vi "Command_TurretControl.vi"(0 "Shooter_Table":dbl[][](array[numeric])=[[55.0, 3350.0, 60.5], [81.0, 3500.0, 54.5], [110.0, 3800.0, 50.5], [143.0, 4100.0, 48.5], [179.0, 4700.0, 47.5], [220.0, 4800.0, 47.5], [250.0, 5800.0, 47.5], [280.0, 5800.0, 45.0]], 3 "Parameters":dbl[](array[numeric]), 6 "Startup":bool) -> (16 "Completed":bool, 17 "Reinit":bool, 20 "Turret_Control_State":T3=enum."No-Op", 21 "Turret_Goal_Angle":dbl, 22 "Camera_Goal_X (deg)":dbl, 23 "Flywheel_Control_State":T2=enum."Speed_Control", 24 "Passive Flywheel Velocity (RPM)":dbl=4000.0, 26 "Cowl_Control_State":T1=enum."No-Op", 27 "Target Cowl Angle (deg)":dbl=52.0)   [LabVIEW 2020]
uses:
  Subsystems/Turret/Turret_States.ctl
  Subsystems/Flywheel/Flywheel_States.ctl
  Subsystems/Cowl/Cowl_States.ctl
  Auto Utilities/Command_Execution_State.ctl
  Globals/Sensor_Values.vi
  Systems/Shooter/Determiner/Shooter_Globals.vi
  Globals/Turret_Globals.vi
panel:
  in  "Shooter_Table 2":dbl[][](array[numeric])=[[55.0, 3350.0, 60.5], [81.0, 3500.0, 54.5], [110.0, 3800.0, 50.5], [143.0, 4100.0, 48.5], [179.0, 4700.0, 47.5], [220.0, 4800.0, 47.5], [250.0, 5800.0, 47.5], [280.0, 5800.0, 45.0]]
  out "angle_to_target":dbl
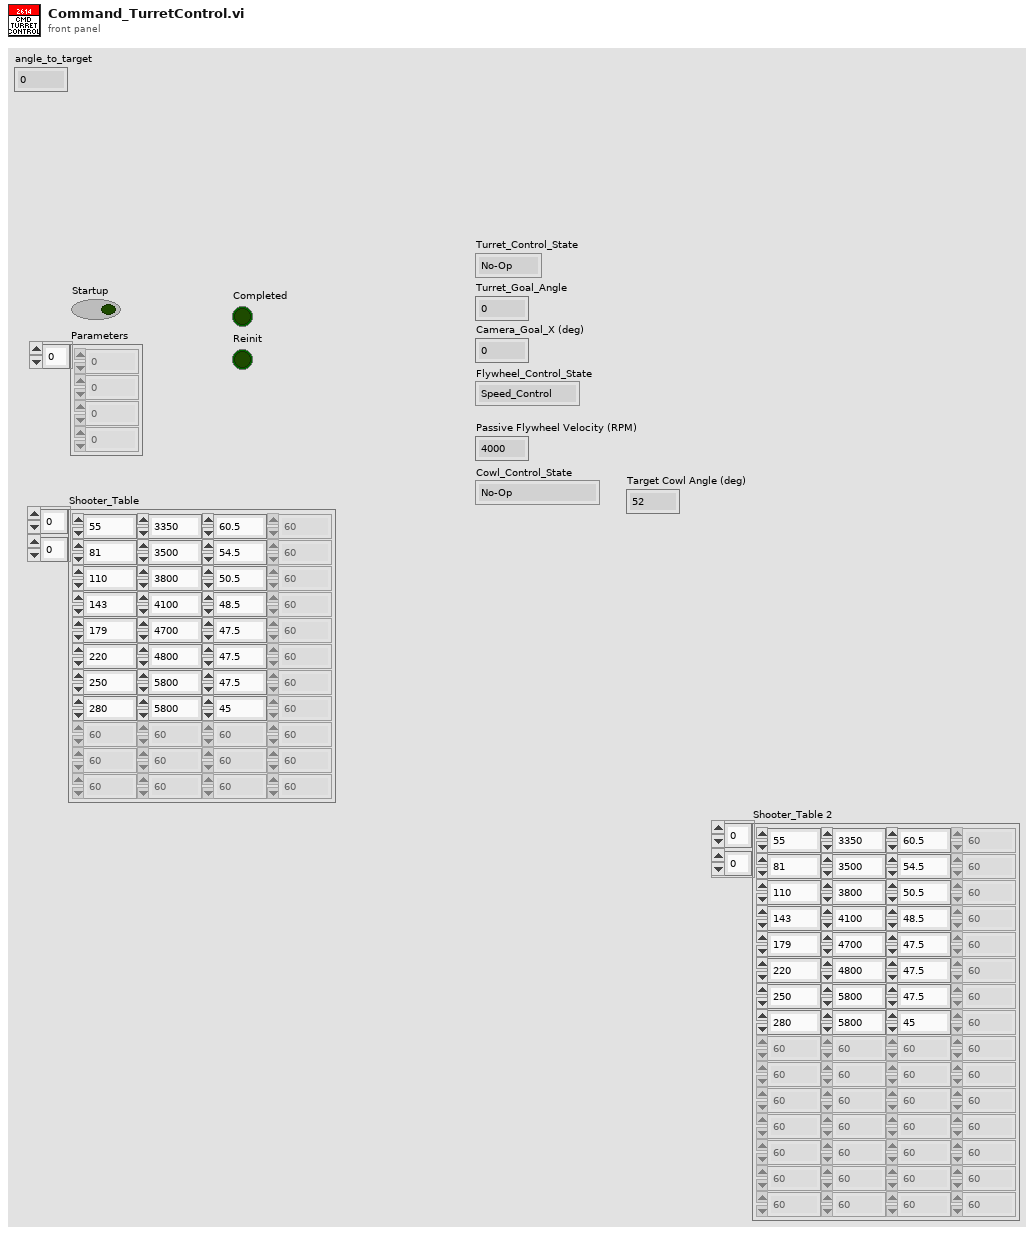
[diagram p1: front panel]
types:
  T1 = typedef "Cowl_States.ctl" = enum16{"Manual_%VBus", "GoToAngle", "No-Op", "GoToZero"}
  T2 = typedef "Flywheel_States.ctl" = enum16{"No-Op", "Percent_Voltage", "Speed_Control", "Speed_Control_Manual", "Command_SpinUp", "Command_SpinUpAuto"}
  T3 = typedef "Turret_States.ctl" = enum16{"Manual_Percent_Voltage", "Target_With_Limelight", "Command_TurnToPosition", "Command_Auto_Target", "GoToZero", "No-Op", "Test_Position_Control", "Position_Control"}
  T4 = typedef "Command_Execution_State.ctl" = enum16{"Initialize", "Execute", "Finish"}
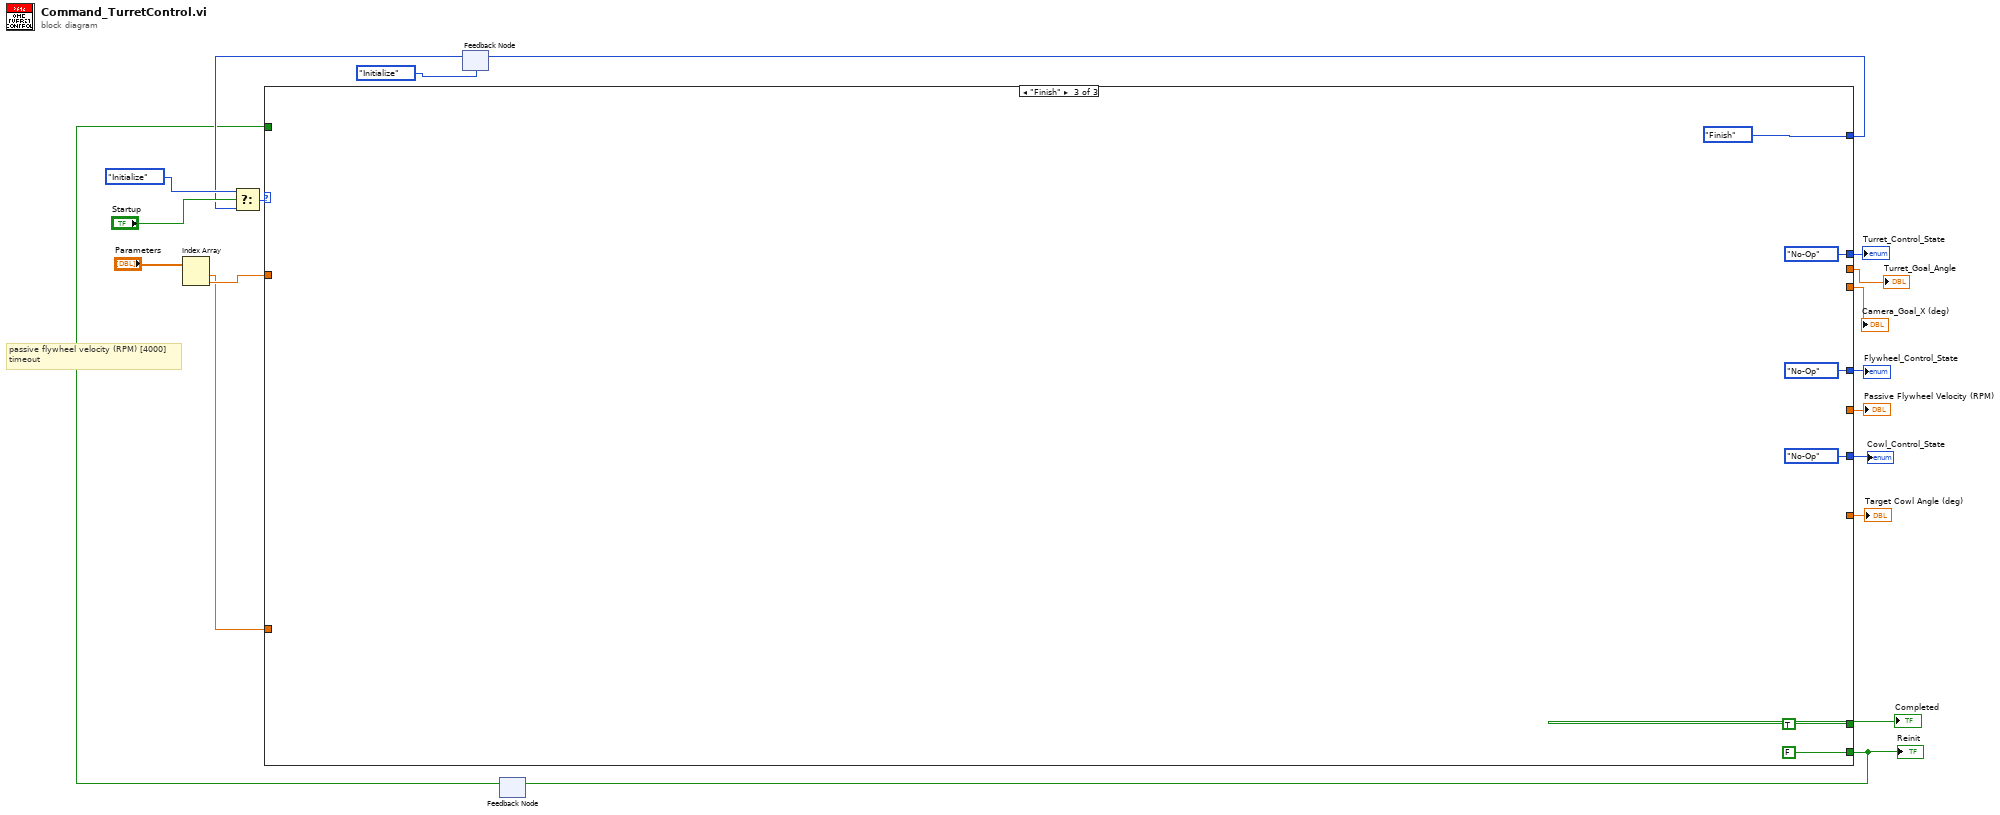
[diagram p0: block diagram]
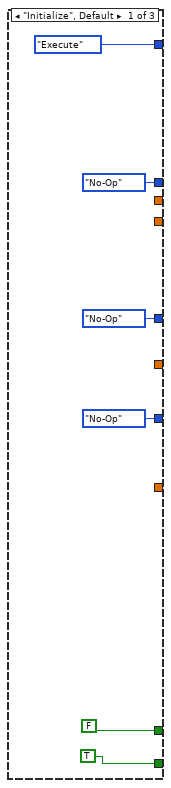
[diagram p2: hidden frame]
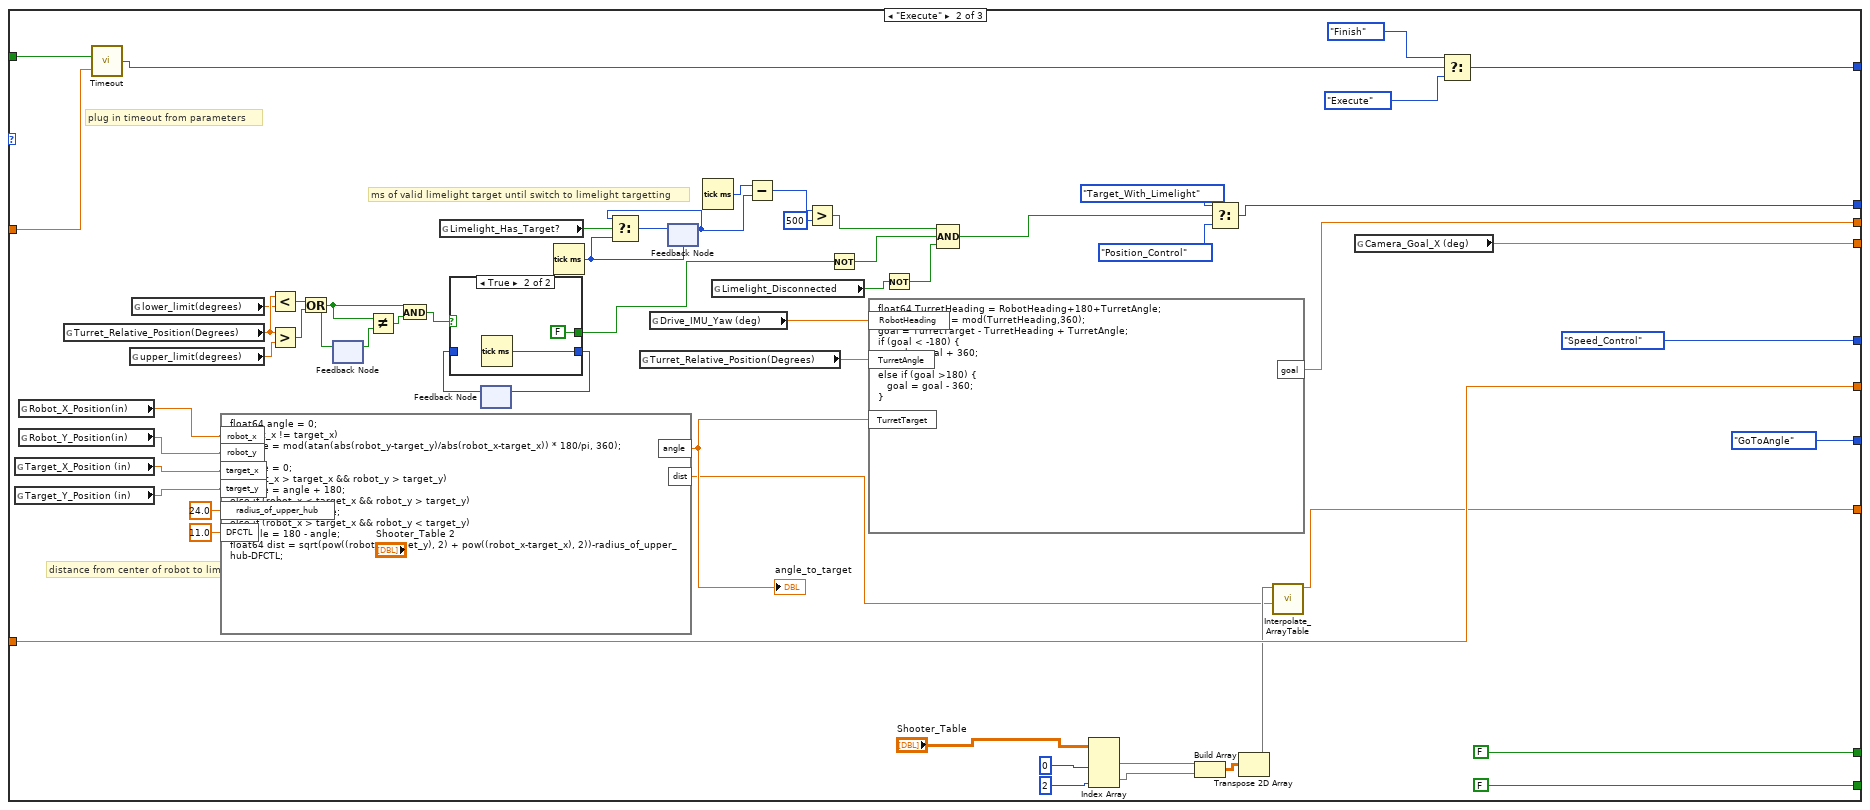
[diagram p3: hidden frame]
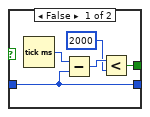
[diagram p4: hidden frame]
diagram:
  # "passive flywheel velocity (RPM) [4000]\ntimeout"
  n1 = Index Array(array="Parameters") -> (element #1=w3:dbl, element #2=w4:dbl)  [unwired: 2 in]
  n2 = feedback #1(Command_Execution_State."Initialize") -> (w15:T4)
  n3 = Select(t=Command_Execution_State."Initialize", s="Startup", f=w15) -> (s? t:f=w17:T4)
  n4 = feedback #2() -> (w11:bool)  [unwired: 1 in]
  n5 = case shown="\"Finish\"" w17 {
    tunnel: [Command_Execution_State."Execute" w81 Command_Execution_State."Finish"] -> w16
    tunnel: [FALSE ("Reinit") FALSE ("Reinit") TRUE ("Reinit")] -> w13
    tunnel: [TRUE ("Reinit") FALSE ("Reinit") FALSE ("Reinit")] -> w12
    tunnel: w11 -> [_ w78 _]
    tunnel: [Turret_States."No-Op" ("Control_State") w48 Turret_States."No-Op" ("Control_State")] -> w9
    tunnel: [_ w47 _] -> w7
    tunnel: [_ w46 _] -> w8
    tunnel: [_ w43 _] -> w6
    tunnel: [Flywheel_States."No-Op" ("Flywheel_Control_State") Flywheel_States."Speed_Control" ("Flywheel_Control_State") Flywheel_States."No-Op" ("Flywheel_Control_State")] -> w5
    tunnel: w4 -> [_ w44 _]
    tunnel: w3 -> [_ w43 _]
    tunnel: [Cowl_States."No-Op" ("Cowl_Control_State") Cowl_States."GoToAngle" ("Cowl_Control_State") Cowl_States."No-Op" ("Cowl_Control_State")] -> w2
    tunnel: [_ w26 _] -> w1
    frame "Initialize", Default {
    }
    frame "Execute" {
      # "distance from center of robot to limelight"
      # "ms of valid limelight target until switch to limelight targetting"
      # "plug in timeout from parameters"
      n6 = global read "Shooter_Globals.vi" "Target_X_Position (in)"() -> (w40:dbl)
      n7 = global read "Shooter_Globals.vi" "Target_Y_Position (in)"() -> (w39:dbl)
      n8 = global read "Sensor_Values.vi" "Robot_X_Position(in)"() -> (w42:dbl)
      n9 = global read "Sensor_Values.vi" "Robot_Y_Position(in)"() -> (w41:dbl)
      n10 = global read "Sensor_Values.vi" "Turret_Relative_Position(Degrees)"() -> (w54:dbl)
      n11 = call "Timeout.vi"("Timeout"=w44, "Initialize"=w78) -> ("Timed Out?"=w77:bool)
      n12 = global read "Turret_Globals.vi" "upper_limit(degrees)"() -> (w52:dbl)
      n13 = global read "Turret_Globals.vi" "lower_limit(degrees)"() -> (w51:dbl)
      n14 = formula code="float64 angle = 0;\nif(robot_x != target_x)\n    angle = mod(atan(abs(robot_y-target_y)/abs(robot_x-target_x)) * 180/pi, 360);\nelse\n    angle = 0;\nif (robot_x > target_x && robot_y > target_y)\n    angle = angle + 180;\nelse if (robot_x < target_x && robot_y > target_y)\n    angle = 360 - angle;\nelse if (robot_x > target_x && robot_y < target_y)\n    angle = 180 - angle;\nfloat64 dist = sqrt(pow((robot_y-target_y), 2) + pow((robot_x-target_x), 2))-radius_of_upper_hub-DFCTL;"("robot_x"=w42, "robot_y"=w41, "target_x"=w40, "target_y"=w39, "radius_of_upper_hub"=24.0 ("input variable"), "DFCTL"=11.0 ("input variable")) -> ("angle"=w36:dbl, "dist"=w28:dbl)
      "angle_to_target" <- w36
      n15 = Less?(x=w54, y=w51) -> (x < y?=w55:bool)
      n16 = Greater?(x=w54, y=w52) -> (0:w53:bool)
      n17 = Or(x=w55, y=w53) -> (x .or. y?=w56:bool)
      n18 = feedback #3() -> (w57:bool)  [unwired: 1 in]
      n19 = feedback-in #3(w56) -> ()
      n20 = Not Equal?(x=w56, y=w57) -> (x != y?=w58:bool)
      n21 = And(x=w56, y=w58) -> (x .and. y?=w59:bool)
      n22 = global read "Sensor_Values.vi" "Limelight_Has_Target?"() -> (w73:bool)
      n23 = feedback #4() -> (w65:u32)  [unwired: 1 in]
      n24 = case shown="True" w59 {
        tunnel: w65 -> [w88 _]
        tunnel: [w88 w90] -> w64
        tunnel: [w87 FALSE] -> w63
        frame False {
          n25 = Tick Count (ms)() -> (millisecond timer value=w85:u32)
          n26 = Subtract(x=w85, y=w88) -> (x-y=w86:u32)
          n27 = Less?(x=w86, y=u32 2000) -> (x < y?=w87:bool)
        }
        frame True {
          n28 = Tick Count (ms)() -> (millisecond timer value=w90:u32)
        }
      }
      n29 = feedback-in #4(w64) -> ()
      n30 = Tick Count (ms)() -> (millisecond timer value=w72:u32)
      n31 = global read "Sensor_Values.vi" "Turret_Relative_Position(Degrees)"() -> (w66:dbl)
      n32 = global read "Sensor_Values.vi" "Drive_IMU_Yaw (deg)"() -> (w67:dbl)
      n33 = feedback #5(w72) -> (w75:u32)
      n34 = Select(t=w75, s=w73, f=w72) -> (s? t:f=w74:u32)
      n35 = feedback-in #5(w74) -> ()
      n36 = Tick Count (ms)() -> (millisecond timer value=w71:u32)
      n37 = global read "Sensor_Values.vi" "Limelight_Disconnected"() -> (w50:bool)
      n38 = Subtract(x=w71, y=w75) -> (x-y=w76:u32)
      n39 = Greater?(x=w76, y=u32 500) -> (0:w60:bool)
      n40 = Not(x=w63) -> (.not. x?=w62:bool)
      n41 = formula code="float64 TurretHeading = RobotHeading+180+TurretAngle;\nTurretHeading = mod(TurretHeading,360);\ngoal = TurretTarget - TurretHeading + TurretAngle;\nif (goal < -180) {\n   goal = goal + 360;\n} \nelse if (goal >180) {\n   goal = goal - 360;\n}"("TurretAngle"=w66, "RobotHeading"=w67, "TurretTarget"=w36) -> ("goal"=w46:dbl)
      n42 = Not(x=w50) -> (.not. x?=w49:bool)
      n43 = Compound Arithmetic op=AND(w60, w62, w49) -> (w61:bool)
      n44 = Index Array(array="Shooter_Table", index (col) #1=0 ("index (row)"), index (col) #2=2 ("index (row)")) -> (element #1=w35:dbl[], element #2=w34:dbl[])  [unwired: 2 in]
      n45 = Build Array(w35, w34) -> (w31:dbl[][])
      n46 = Select(t=Turret_States."Target_With_Limelight" ("Control_State"), s=w61, f=Turret_States."Position_Control" ("Control_State")) -> (s? t:f=w48:T3)
      n47 = Transpose 2D Array(2D array=w31) -> (transposed array=w30:dbl[][])
      n48 = call "Interpolate_ArrayTable.vi"("Desired_Distance"=w28, "array"=w30) -> ("RPM"=w26:dbl)  [unwired: 9 in]
      n49 = global read "Sensor_Values.vi" "Camera_Goal_X (deg)"() -> (w47:dbl)
      n50 = Select(t=Command_Execution_State."Finish", s=w77, f=Command_Execution_State."Execute") -> (s? t:f=w81:T4)
    }
    frame "Finish" {
    }
  }
  "Reinit" <- w12
  "Completed" <- w13
  "Turret_Control_State" <- w9
  "Turret_Goal_Angle" <- w8
  "Camera_Goal_X (deg)" <- w7
  "Passive Flywheel Velocity (RPM)" <- w6
  "Flywheel_Control_State" <- w5
  "Cowl_Control_State" <- w2
  "Target Cowl Angle (deg)" <- w1
  n51 = feedback-in #1(w16) -> ()
  n52 = feedback-in #2(w12) -> ()
